vi "JYMoveMono.vi"(8 "error in (no error)":errorcluster, 10 "?":dbl, 11 "JYMONOLib.IJYMonoReqd":refnum<k7>) -> (0 "error out":errorcluster)   [LabVIEW 2017]
doc: "JYMoveToWavelength.vi\n\nMoves the mono to a new wavelength.\n\nInputs\nMono RefNum - the LabView automation refnum of the mono\nTarget Wavelength - double; new wavelength for mono\nError Cluster\n\n\nOutputs\nMonoRefNum - the LabView automation refnum is supplied as\n an output\nError Cluster"
panel:
  # "Enter a value in the target wavelength\ncontrol and press the Enter key to move\nthe mono.  Click the OK button to Exit"
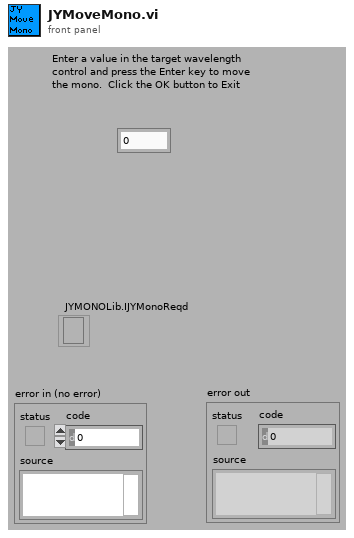
[diagram p1: front panel]
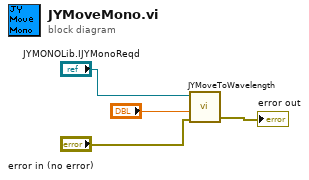
[diagram p0: block diagram]
diagram:
  n1 = call "JYMoveToWavelength.vi"("error in (no error)"="error in (no error)", "Target WL"="?", "RefNum In"="JYMONOLib.IJYMonoReqd") -> ("error out"=→"error out":errorcluster)  [unwired: 1 in, 2 out]
